vi "Celsius Temperature Simulator.vi"(11 "entrée d'erreur (pas d'erreur)":errorcluster) -> (4 "Température":dbl, 15 "sortie d'erreur":errorcluster)   [LabVIEW 2009]
doc: "Génère une température aléatoire simulée entre 20 et 30 degrés Celsius."
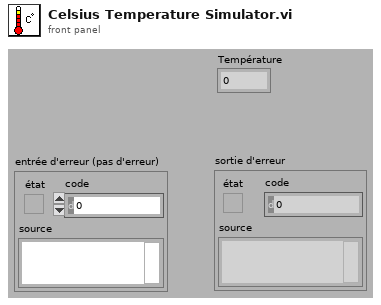
[diagram p1: front panel]
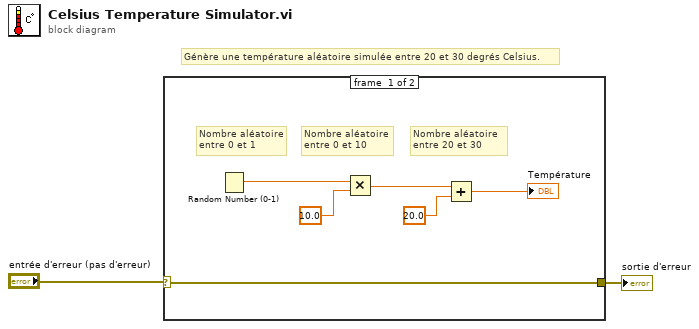
[diagram p0: block diagram]
diagram:
  # "Génère une température aléatoire simulée entre 20 et 30 degrés Celsius."
  n1 = case "Structure Condition" shown="Pas d'erreur" "entrée d'erreur (pas d'erreur)" {
    selector: "entrée d'erreur (pas d'erreur)" -> [w3 w9]
    tunnel: [w3 w9] -> w1
    frame #0 {
      # "Nombre aléatoire entre 20 et 30"
      # "Nombre aléatoire entre 0 et 10"
      # "Nombre aléatoire entre 0 et 1"
      n2 = Random Number (0-1) ("Nombre aléatoire (0-1)")() -> (number: 0 to 1=w8:dbl)
      n3 = Multiply ("Multiplier")(x=w8, y=10.0) -> (x*y=w6:dbl)
      n4 = Add ("Additionner")(x=w6, y=20.0) -> (x+y=→"Température":dbl)
    }
    frame #1 {
    }
  }
  "sortie d'erreur" <- w1
